vi "Query Alarm Condition.vi"(8 "error in (no error)":errorcluster, 10 "Channel (1:1)":u16(ring)=1 items=["1"=1, "2"=2, "3"=3, "4"=4, "5"=5, "6"=6, "7"=7, "8"=8, "9"=9, "10"=10, "11"=11, "12"=12, "13"=13, "14"=14, "15"=15, "16"=16, "A (Control Input)"=17], 11 "VISA resource name":refnum<visa-resource-name>) -> (0 "error out":errorcluster, 1 "Alarm Low Status":bool, 2 "Alarm High Status":bool, 3 "VISA resource name out":refnum<visa-resource-name>)   [LabVIEW 2015, in "Lake Shore 372.lvlib"]
doc: "Queries the status of the alarm for the selected channel."
uses:
  <instrlib>/Lake Shore 372/Lake Shore 372.lvlib
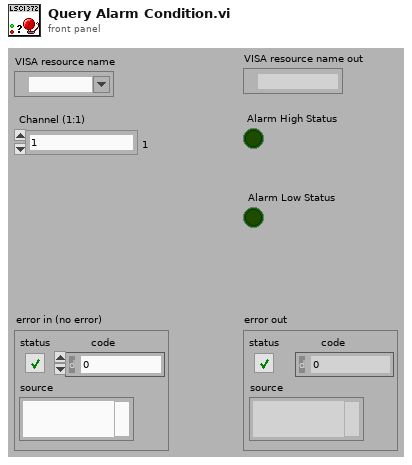
[diagram p1: front panel]
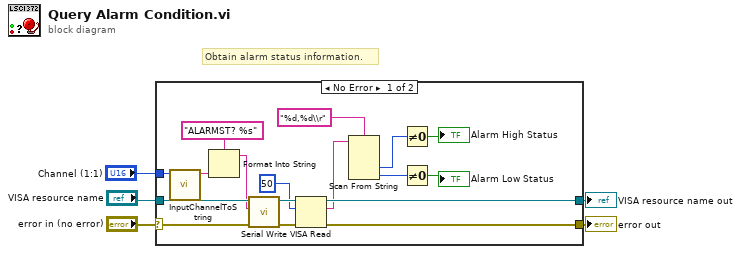
[diagram p0: block diagram]
diagram:
  # "Obtain alarm status information."
  n1 = case shown="No Error" "error in (no error)" {
    selector: "error in (no error)" -> [w6 w23]
    tunnel: "VISA resource name" -> [w17 w24]
    tunnel: [w16 w24] -> w4
    tunnel: [w15 w23] -> w3
    tunnel: "Channel (1:1)" -> [w8 _]
    frame No Error {
      n2 = call <instrlib>:"InputChannelToString.vi"("Channel (1)"=w8) -> ("Channel Str"=w7:string)  [unwired: 10 in]
      n3 = Format Into String(format string="ALARMST? %s", w7) -> (resulting string=w13:string)  [unwired: 2 in, 1 out]
      n4 = call <instrlib>:"Serial Write.vi"("error in (no error)"=w6, "Write Buffer (\"\")"=w13, "VISA resource name"=w17) -> ("error out"=w21:errorcluster, "VISA resource name out"=w22:refnum<visa-resource-name>)  [unwired: 6 in, 1 out]
      n5 = VISA Read(VISA resource name=w22, byte count=50, error in (no error)=w21) -> (VISA resource name out=w16:refnum<visa-resource-name>, read buffer=w11:string, error out=w15:errorcluster)  [unwired: 1 out]
      n6 = Scan From String(format string="%d,%d\\r", input string=w11) -> (output 1=w10:i32, output 2=w9:i32)  [unwired: 4 in, 3 out]
      n7 = Not Equal To 0?(x=w10) -> (x != 0?=→"Alarm High Status":bool)
      n8 = Not Equal To 0?(x=w9) -> (x != 0?=→"Alarm Low Status":bool)
    }
    frame Error {
    }
  }
  "error out" <- w3
  "VISA resource name out" <- w4
